vi "parse fifo value.vi"(11 "Element":u32) -> (0 "data":u8, 1 "index":u8, 2 "device":u8, 3 "action":T1, 5 "full element":u32)   [LabVIEW 2013]
uses:
  profibus master action.ctl
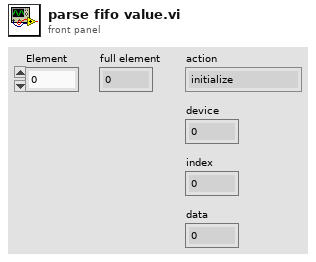
[diagram p1: front panel]
types:
  T1 = typedef "profibus master action.ctl" = enum8{"initialize", "uninitialize", "stop", "set input", "get input", "get input size", "set output", "get output", "get output size", "get diagnostic", "transfer data", "transfer diagnostics"}
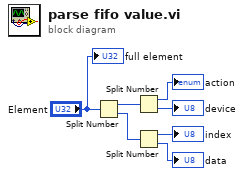
[diagram p0: block diagram]
diagram:
  n1 = Split Number(x="Element") -> (hi(x)=w6:u16, lo(x)=w5:u16)
  n2 = Split Number(x=w6) -> (hi(x)=→"action":u8, lo(x)=→"device":u8)
  n3 = Split Number(x=w5) -> (hi(x)=→"index":u8, lo(x)=→"data":u8)
  "full element" <- "Element"
